vi "Agilent N934X Series Acquire Measurement.vi"() -> ()   [LabVIEW 2022 SP3]
doc: "This example shows how to configure the spectrum analyzer to acquire measurement."
uses:
  <instrlib>/Agilent N934X Series/Agilent N934X Series.lvlib
panel:
  out "Channel Power Density (dBm/Hz)":dbl
  out "Channel Power (dBm/Integrated BW MHz)":dbl
  in  "Averaging Type (0: Log Power)":i32(ring) items=["Log Power", "Power", "Voltage"]
  in  "Average Count (100)":i32=100
  in  "Reference Level Offset (0 dB)":dbl
  in  "Reference Level (0 dBm)":i32
  in  "Frequency Span (7 GHz)":dbl=7000000000.0
  in  "Center Frequency (3.5 GHz)":dbl=3500000000.0
  in  "VISA resource name":refnum<visa-resource-name>
  # "(c) 2012 - 2025 National Instruments.  ALL RIGHTS RESERVED."
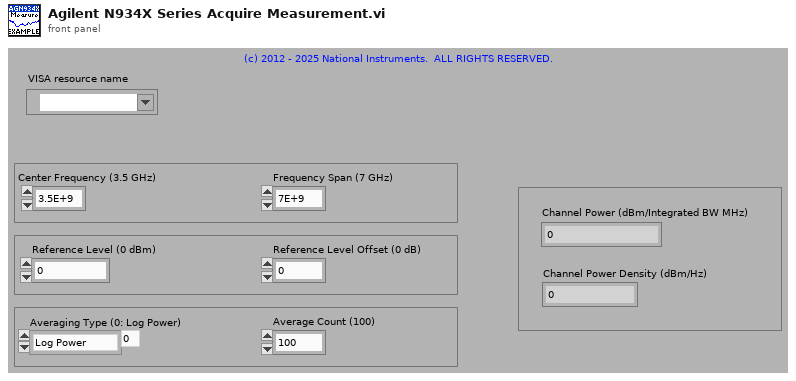
[diagram p1: front panel]
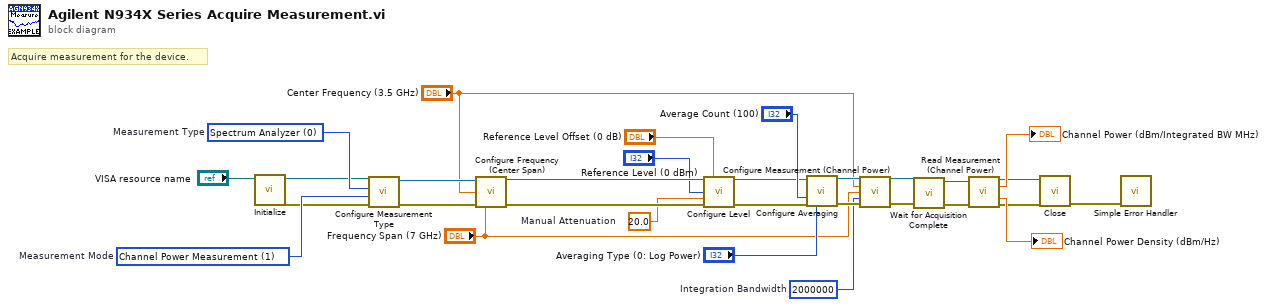
[diagram p0: block diagram]
diagram:
  w1 = 20.0  # Manual Attenuation
  w4 = 2000000  # Integration Bandwidth
  w15 = 1 items=["Off", "Channel Power Measurement", "Adjacent Channel Power Ratio Measurement", "Occupied Bandwidth Measurement", "Spectrum Monitor"]  # Measurement Mode
  w29 = 0 items=["Spectrum Analyzer", "Tracking Generator", "Power Meter"]  # Measurement Type
  # "Acquire measurement for the device."
  n1 = call <instrlib>:"Initialize.vi"("VISA resource name"="VISA resource name") -> ("error out"=w11:errorcluster, "VISA resource name out"=w12:refnum<visa-resource-name>)  [unwired: 9 in]
  n2 = call <instrlib>:"Configure Measurement Type.vi"("error in (no error)"=w11, "Measurement Mode (0: Off)"=w15, "Measurement Type (0: Spectrum Analyzer)"=w29, "VISA resource name"=w12) -> ("error out"=w27:errorcluster, "VISA resource name out"=w28:refnum<visa-resource-name>)  [unwired: 6 in]
  n3 = call <instrlib>:"Configure Frequency (Center Span).vi"("VISA resource name"=w28, "Center Frequency (3.5E+9 Hz)"="Center Frequency (3.5 GHz)", "error in (no error)"=w27, "Frequency Span (7E+9 Hz)"="Frequency Span (7 GHz)") -> ("VISA resource name out"=w26:refnum<visa-resource-name>, "error out"=w25:errorcluster)  [unwired: 10 in]
  n4 = call <instrlib>:"Configure Level.vi"("VISA resource name"=w26, "Reference Level Offset (0 dB)"="Reference Level Offset (0 dB)", "Reference Level (0 dBm)"="Reference Level (0 dBm)", "Manual Attenuation (20 dB)"=w1, "error in (no error)"=w25) -> ("VISA resource name out"=w14:refnum<visa-resource-name>, "error out"=w13:errorcluster)  [unwired: 9 in]
  n5 = call <instrlib>:"Configure Averaging.vi"("VISA resource name"=w14, "Average Count (100)"="Average Count (100)", "error in (no error)"=w13, "Averaging Type (0: Log Power)"="Averaging Type (0: Log Power)") -> ("VISA resource name out"=w22:refnum<visa-resource-name>, "error out"=w21:errorcluster)  [unwired: 10 in]
  n6 = call <instrlib>:"Configure Measurement (Channel Power).vi"("VISA resource name"=w22, "Integration Bandwidth (2E+6 Hz)"="Center Frequency (3.5 GHz)", "Channel Power Span (3E+6 Hz)"="Frequency Span (7 GHz)", "Center Frequency (3.5E+9 Hz)"=w4, "error in (no error)"=w21) -> ("VISA resource name out"=w10:refnum<visa-resource-name>, "error out"=w9:errorcluster)  [unwired: 9 in]
  n7 = call <instrlib>:"Wait for Acquisition Complete.vi"("error in (no error)"=w9, "VISA resource name"=w10) -> ("error out"=w7:errorcluster, "VISA resource name out"=w8:refnum<visa-resource-name>)  [unwired: 8 in]
  n8 = call <instrlib>:"Read Measurement (Channel Power).vi"("VISA resource name"=w8, "error in (no error)"=w7) -> ("VISA resource name out"=w18:refnum<visa-resource-name>, "Channel Power(dBm/Integrated BW MHz)"=→"Channel Power (dBm/Integrated BW MHz)":dbl, "Channel Power Density(dBm/Hz)"=→"Channel Power Density (dBm/Hz)":dbl, "error out"=w17:errorcluster)  [unwired: 10 in]
  n9 = call <instrlib>:"Close.vi"("error in (no error)"=w17, "VISA resource name"=w18) -> ("error out"=w16:errorcluster)  [unwired: 9 in]
  n10 = call <vilib>:"Simple Error Handler.vi"("error in (no error)"=w16) -> ()  [unwired: 4 in, 5 out]
